vi "FileWriteTestRT.vi"() -> ()   [LabVIEW 2017]
uses:
  State.ctl
panel:
  out "Log File Path":path=path "c:/ni-rt/LabVIEW Data/Test17"
  in  "Log File Name":string="Test17"
  out "Write Test Folder":path=path "c:/ni-rt/LabVIEW Data/MyDataFolder1/1/7"
  out "Write Iterations":i32=111
  in  "Iterations":i64=1000
  in  "Files Written Per Iteration":i32=5
  out "Elapsed Time This Iteration (ms)":u32=8
  out "error out":errorcluster
  in  "Folder Path: c:\\ni-rt\\LabVIEW Data\\...":string="MyDataFolder1\\1\\7"
  in  "stop":bool
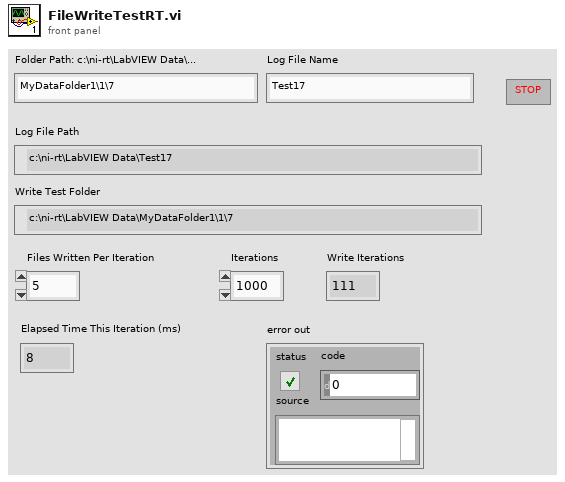
[diagram p1: front panel]
types:
  T1 = cluster{"File Write Test Path":path, "Write Time per File":dbl, "Write Iterations":i32, "Write Time (ms)":u32, "Stop":bool, "Log File Ref":refnum<k34>}
  T2 = typedef "State.ctl" = enum16{"Initialize", "Write", "Log", "Stop"}
  T3 = enum16{"open", "open or create", "create or replace", "create", "open (read-only)"}
  T4 = enum16{"open", "replace", "create", "open or create", "replace or create", "replace or create with confirmation"}
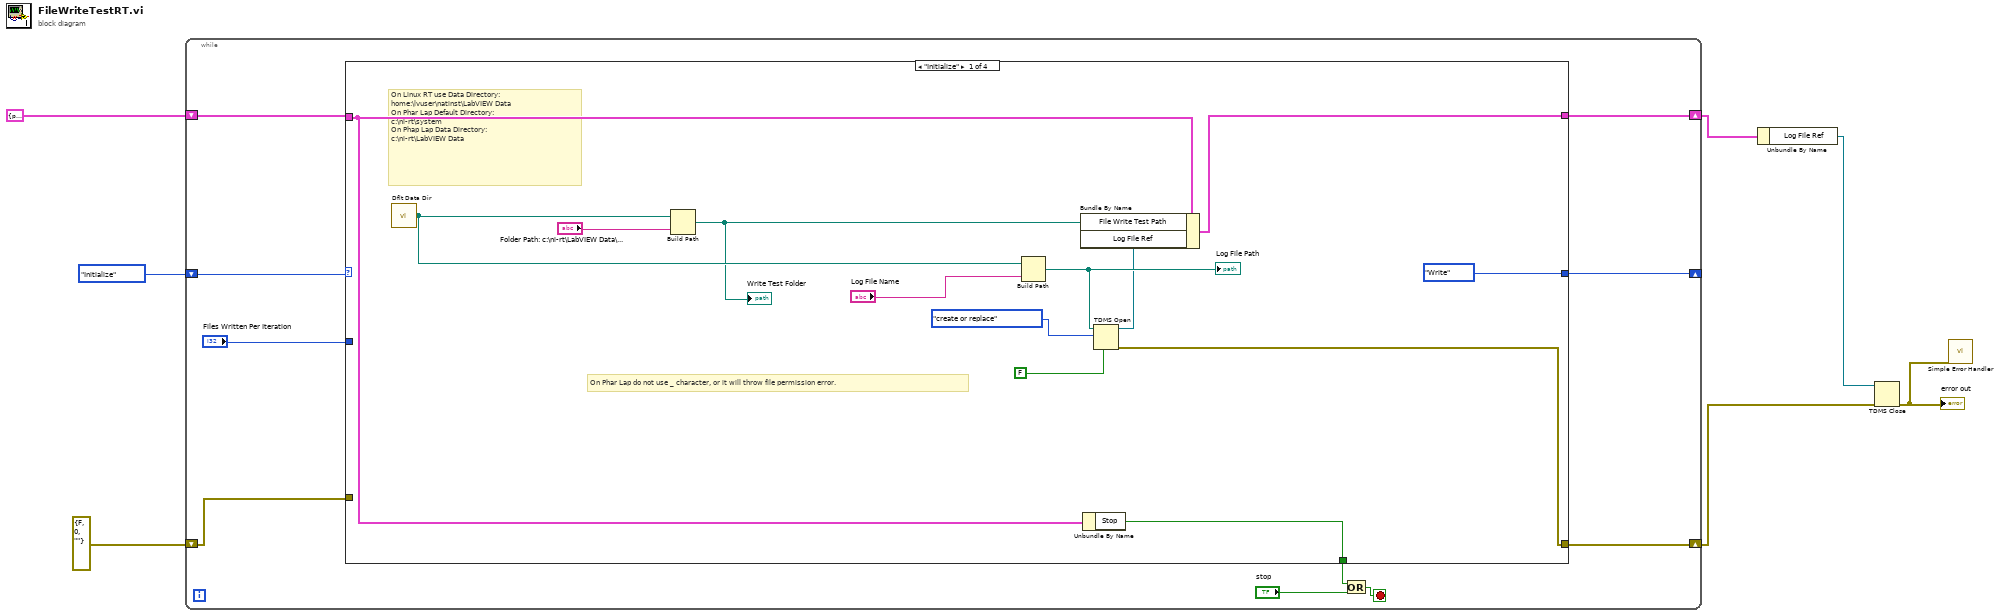
[diagram p0: block diagram]
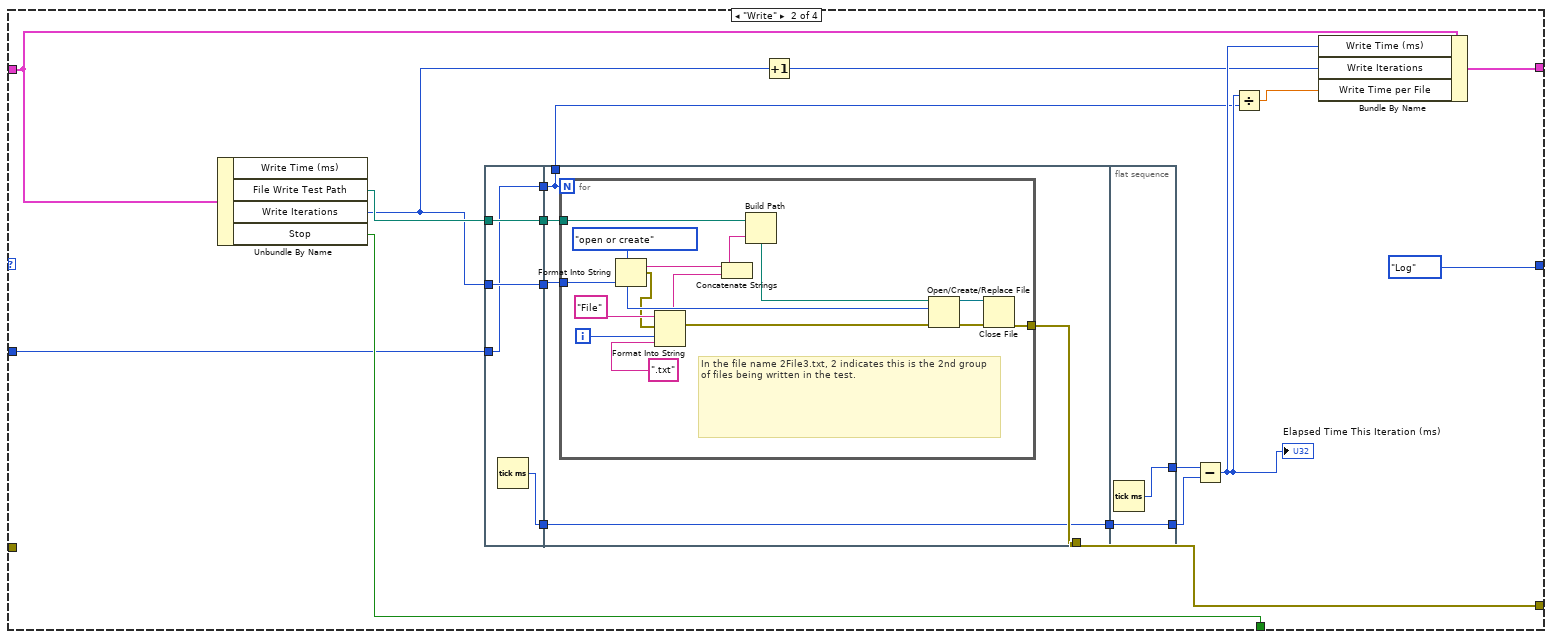
[diagram p2: hidden frame]
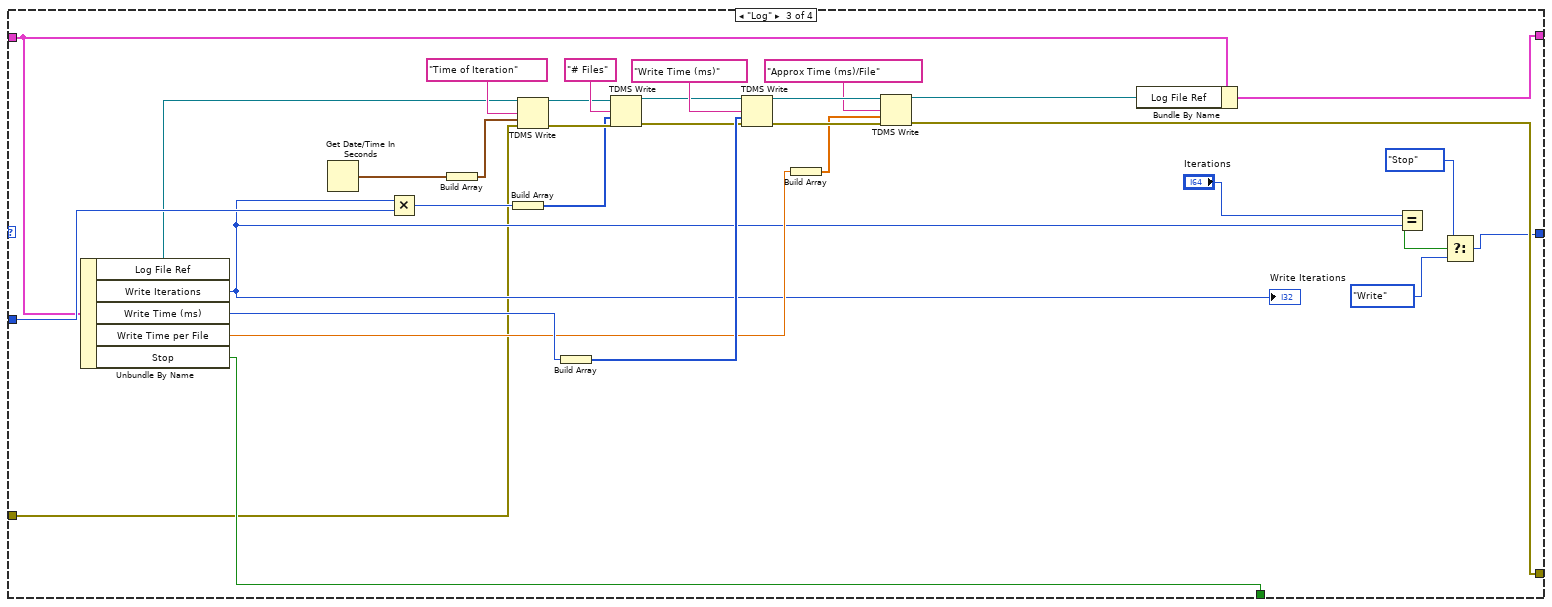
[diagram p3: hidden frame]
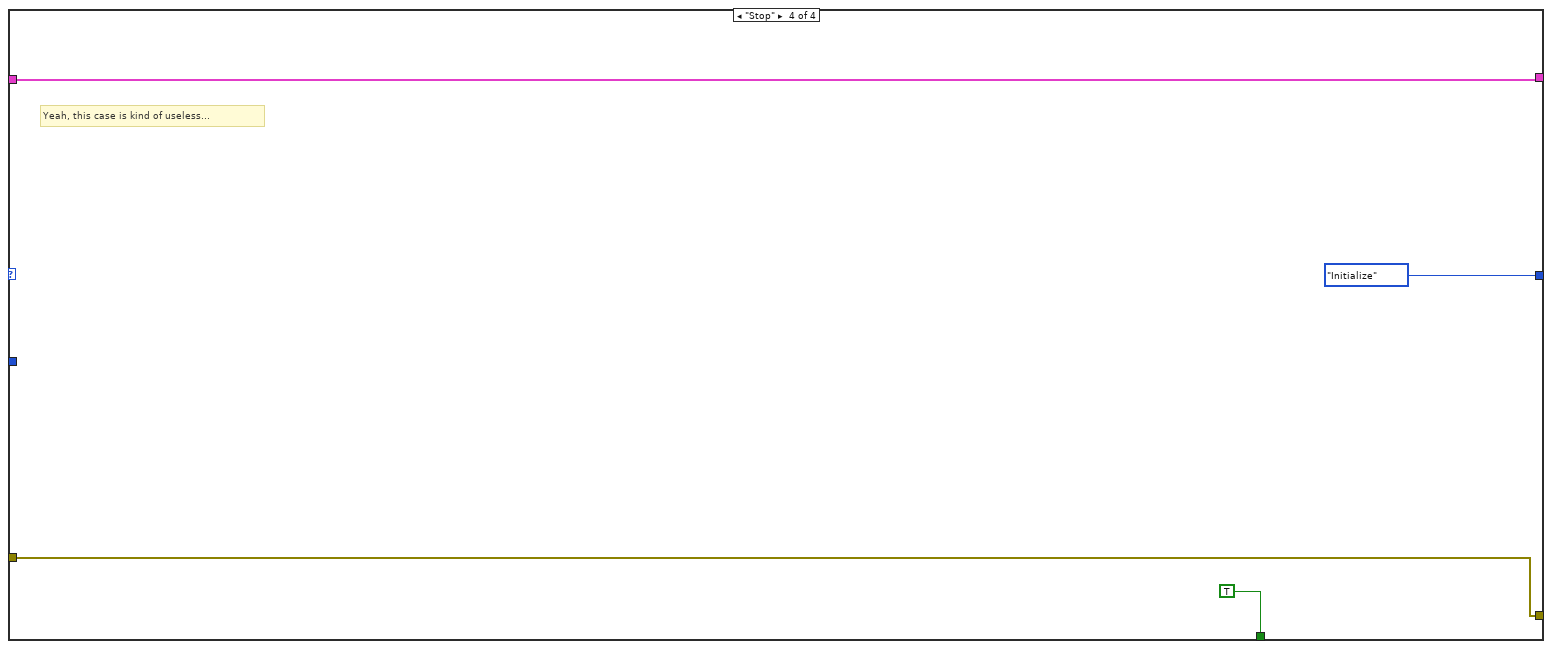
[diagram p4: hidden frame]
diagram:
  n1 = while {
    shift-right: [w14] -> _
    shift-left: State."Initialize" -> [w17]
    shift-right: [w16] -> w2
    shift-left: errorcluster {"status"=FALSE, "code"=0, "source"=""} ("error out") -> [w15]
    shift-right: [w9] -> w4
    shift-left: T1 {"File Write Test Path"=path "", "Write Time per File"=0.0, "Write Iterations"=0, "Write Time (ms)"=0, "Stop"=FALSE, "Log File Ref"=refnum} -> [w10]
    stop <- w11 stop-if-true
    n2 = case shown="\"Initialize\"" w17 {
      tunnel: [w20 w49 w95 w108] -> w16
      tunnel: w15 -> [_ _ w80 w108]
      tunnel: [State."Write" State."Log" w90 State."Initialize"] -> w14
      tunnel: [w26 w38 w81 TRUE] -> w13
      tunnel: w10 -> [w27 w42 w78 w109]
      tunnel: [w28 w41 w76 w109] -> w9
      tunnel: "Files Written Per Iteration" -> [_ w32 w87 _]
      frame "Initialize" {
        # "On Phar Lap do not use _ character, or it will throw file permission error."
        # "On Linux RT use Data Directory:\nhome:\\lvuser\\natinst\\LabVIEW Data\nOn Phar Lap Default Directory:\nc:\\ni-rt\\system\nOn Phap Lap Data Directory:\nc:\\ni-rt\\LabVIEW Data"
        n3 = call <vilib>:"Dflt Data Dir.vi"() -> ("App:Default Data Directory"=w19:path)
        n4 = Build Path(base path=w19, name or relative path="Folder Path: c:\\ni-rt\\LabVIEW Data\\...") -> (appended path=w18:path)
        "Write Test Folder" <- w18
        n5 = Build Path(base path=w19, name or relative path="Log File Name") -> (appended path=w22:path)
        "Log File Path" <- w22
        n6 = Unbundle By Name(w27) -> ("Stop"=w26:bool)
        n7 = TDMS Open(6:FALSE ("disable buffering (T)"), 10:T3."create or replace" ("operation"), 11:w22) -> (0:w20:errorcluster, 3:w21:refnum<k34>)  [unwired: 4 in]
        n8 = Bundle By Name(cluster=w27, "File Write Test Path"=w18, "Log File Ref"=w21) -> (w28:T1)
      }
      frame "Write" {
        n9 = Unbundle By Name(w42) -> ("File Write Test Path"=w40:path, "Write Iterations"=w39:i32, "Stop"=w38:bool)  [unwired: 1 out]
        n10 = flat-sequence {
          tunnel: w40 -> [w53]
          tunnel: [w53] -> w47
          tunnel: [w50] -> w46
          tunnel: w39 -> [w52]
          tunnel: [w52] -> w44
          tunnel: [w51] -> w36
          tunnel: w32 -> [w50]
          tunnel: [w58] -> w49
          tunnel: w47 -> [w57]
          tunnel: w46 -> [w54]
          tunnel: w44 -> [w56]
          tunnel: w36 -> [w55]
          tunnel: [w55] -> w34
          tunnel: [w54] -> w31
          tunnel: [w75] -> w35
          tunnel: w34 -> [w74]
          tunnel: [w74] -> w33
          frame #0 {
            n11 = Tick Count (ms)() -> (millisecond timer value=w51:u32)
          }
          frame #1 {
            n12 = for {
              N: w54 -> [_]
              tunnel: [w66] -> w58
              tunnel: w56 -> [w62]
              tunnel: w57 -> [w59]
              i -> [w72]
              # "In the file name 2File3.txt, 2 indicates this is the 2nd group of files being written in the test."
              n13 = Format Into String(w62) -> (resulting string=w61:string, error out=w60:errorcluster)  [unwired: 3 in]
              n14 = Format Into String(initial string="File", error in=w60, w72, ".txt") -> (resulting string=w64:string, error out=w70:errorcluster)  [unwired: 1 in]
              n15 = Concatenate Strings(w61, w64) -> (w65:string)
              n16 = Build Path(base path=w59, name or relative path=w65) -> (appended path=w69:path)
              n17 = Open/Create/Replace File(file path (use dialog)=w69, error in=w70, operation (0:open)=T4."open or create") -> (refnum out=w68:refnum<file>, error out=w67:errorcluster)  [unwired: 3 in, 1 out]
              n18 = Close File(refnum=w68, error in=w67) -> (error out=w66:errorcluster)  [unwired: 1 out]
            }
          }
          frame #2 {
            n19 = Tick Count (ms)() -> (millisecond timer value=w75:u32)
          }
        }
        n20 = Increment(x=w39) -> (x+1=w43:i32)
        n21 = Subtract(x=w35, y=w33) -> (x-y=w45:u32)
        "Elapsed Time This Iteration (ms)" <- w45
        n22 = Divide(x=w45, y=w31) -> (x/y=w37:dbl)
        n23 = Bundle By Name(cluster=w42, "Write Time (ms)"=w45, "Write Iterations"=w43, "Write Time per File"=w37) -> (w41:T1)
      }
      frame "Log" {
        n24 = Unbundle By Name(w78) -> ("Log File Ref"=w79:refnum<k34>, "Write Iterations"=w82:i32, "Write Time (ms)"=w86:u32, "Write Time per File"=w84:dbl, "Stop"=w81:bool)
        "Write Iterations" <- w82
        n25 = Get Date/Time In Seconds() -> (seconds since 1Jan1904=w106:timestamp)
        n26 = Multiply(x=w82, y=w87) -> (x*y=w88:i32)
        n27 = Build Array(w106) -> (w105:timestamp[])
        n28 = Build Array(w88) -> (w89:i32[])
        n29 = TDMS Write(0:w79, 7:"Time of Iteration", 9:w105, 11:w80) -> (4:w101:refnum<k34>, 15:w98:errorcluster)  [unwired: 2 in, 2 out]
        n30 = Build Array(w86) -> (w103:u32[])
        n31 = TDMS Write(0:w101, 7:"# Files", 9:w89, 11:w98) -> (4:w100:refnum<k34>, 15:w97:errorcluster)  [unwired: 2 in, 2 out]
        n32 = TDMS Write(0:w100, 7:"Write Time (ms)", 9:w103, 11:w97) -> (4:w99:refnum<k34>, 15:w96:errorcluster)  [unwired: 2 in, 2 out]
        n33 = Build Array(w84) -> (w83:dbl[])
        n34 = TDMS Write(0:w99, 7:"Approx Time (ms)/File", 9:w83, 11:w96) -> (4:w77:refnum<k34>, 15:w95:errorcluster)  [unwired: 2 in, 2 out]
        n35 = Bundle By Name(cluster=w78, "Log File Ref"=w77) -> (w76:T1)
        n36 = Equal?(x="Iterations", y=w82) -> (x = y?=w93:bool)
        n37 = Select(t=State."Stop", s=w93, f=State."Write") -> (s? t:f=w90:T2)
      }
      frame "Stop" {
        # "Yeah, this case is kind of useless..."
      }
    }
    n38 = Compound Arithmetic op=OR(w13, "stop") -> (w11:bool)
  }
  n39 = Unbundle By Name(w4) -> ("Log File Ref"=w3:refnum<k34>)
  n40 = TDMS Close(8:w2, 11:w3) -> (0:w1:errorcluster)  [unwired: 1 out]
  "error out" <- w1
  n41 = call <vilib>:"Simple Error Handler.vi"("error in (no error)"=w1) -> ()  [unwired: 4 in, 5 out]
